vi "6b.vi"(11 "f":dbl) -> (3 "Array":dbl[](array[numeric]))   [LabVIEW 2016]
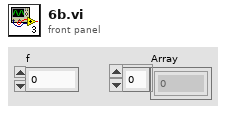
[diagram p1: front panel]
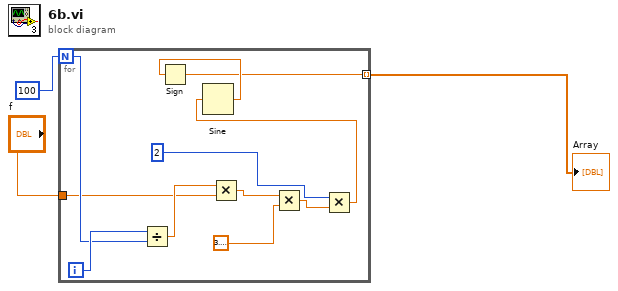
[diagram p0: block diagram]
diagram:
  n1 = for {
    N: 100 -> [w13]
    tunnel: "f" -> [w11]
    tunnel: [w4] -> w3 mode=indexing
    i -> [w14]
    n2 = Divide(x=w14, y=w13) -> (x/y=w12:dbl)
    n3 = Multiply(x=w12, y=w11) -> (x*y=w9:dbl)
    n4 = Multiply(x=w9, y=3.141592653589793) -> (x*y=w7:dbl)
    n5 = Multiply(x=2, y=w7) -> (x*y=w6:dbl)
    n6 = Sine(x=w6) -> (sin(x)=w5:dbl)
    n7 = Sign(1:w5) -> (0:w4:dbl)
  }
  "Array" <- w3
